vi "Launch State Update Metronome.vi"(8 "error in (no error)":errorcluster, 10 "Status Update Period [1000 ms]":i32=1000, 11 "Actor in":refnum<class "Actor.lvclass">) -> (0 "error out":errorcluster, 3 "Actor out":refnum<class "Actor.lvclass">)   [LabVIEW 2015, in "Actor.lvclass"]
uses:
  Actor.lvclass
  Actor.lvclass/Actor.ctl
  Metronome/Actor/Metronome Actor.lvclass
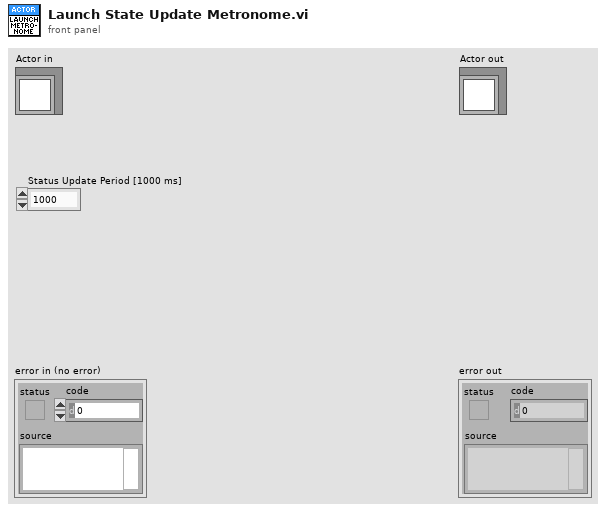
[diagram p1: front panel]
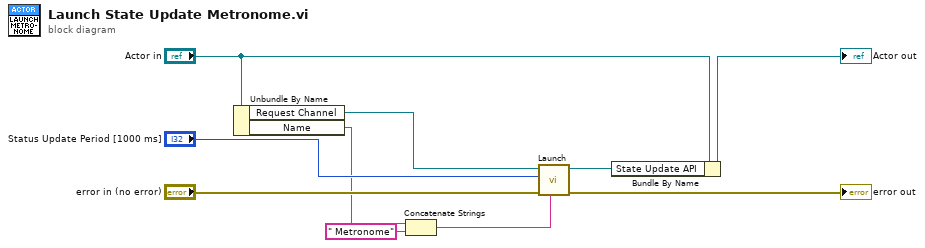
[diagram p0: block diagram]
diagram:
  n1 = Unbundle By Name("Actor in") -> ("Request Channel"=w8:refnum<class "Messenger.lvclass">, "Name"=w3:string)
  n2 = Concatenate Strings(w3, " Metronome" ("string")) -> (w1:string)
  n3 = call "Launch.vi"("Name"=w1, "error in (no error)"="error in (no error)", "Period [ms]"="Status Update Period [1000 ms]", "Response Channel"=w8) -> ("error out"=→"error out":errorcluster, "Actor API"=w10:refnum<class "Metronome Actor API.lvclass">)  [unwired: 6 in]
  n4 = Bundle By Name(cluster="Actor in", "State Update API"=w10) -> (→"Actor out":refnum<class "Actor.lvclass">)
